vi "边沿计数_事件导出.vi"() -> ()   [LabVIEW 2013]
doc: "This example demonstrates how to count the pulse's edges."
uses:
  <userlib>/ArtDAQ/_SubVI/ArtDAQ_CreateCICountEdgesChan.vi
  <userlib>/ArtDAQ/_SubVI/ArtDAQ_CfgSampClkTiming.vi
  <userlib>/ArtDAQ/_SubVI/ArtDAQ_Read Counter U32 NSamp.vi
panel:
  in  "输出端口":string="Dev1/CTR0"
  in  "脉冲输出极性":i32(ring)=10095 items=["高电平"=10095, "低电平"=10096]
  in  "反转空闲状态":i32(ring)=10192 items=["高"=10192, "低"=10214]
  in  "输出方式":i32(ring)=10265 items=["脉冲方式"=10265, "反转方式"=10307]
  in  "每通道点数":i32=100
  in  "采样速率":dbl=1000.0 format="%#_13g"
  in  "时钟源":string="/Dev1/PFI3"
  in  "计数器":string="Dev1/CTR0"
  out "数据":u32[](array[numeric])
  in  "停止":bool
  out "错误输出":errorcluster
  # "通道属性"
  # "输出事件"
  # "定时"
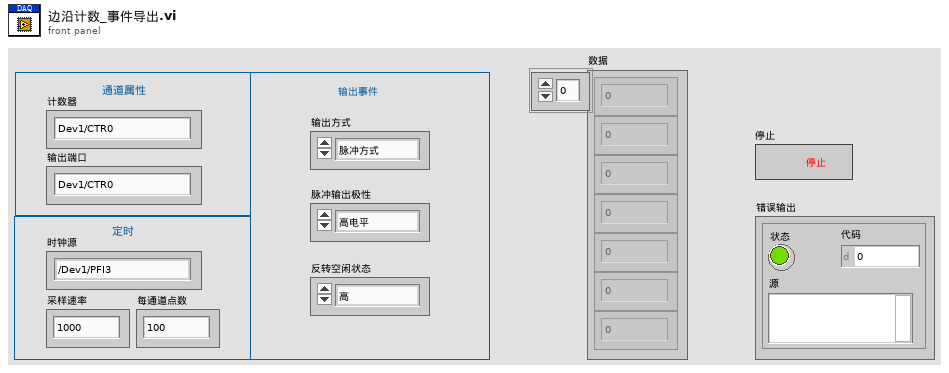
[diagram p1: front panel]
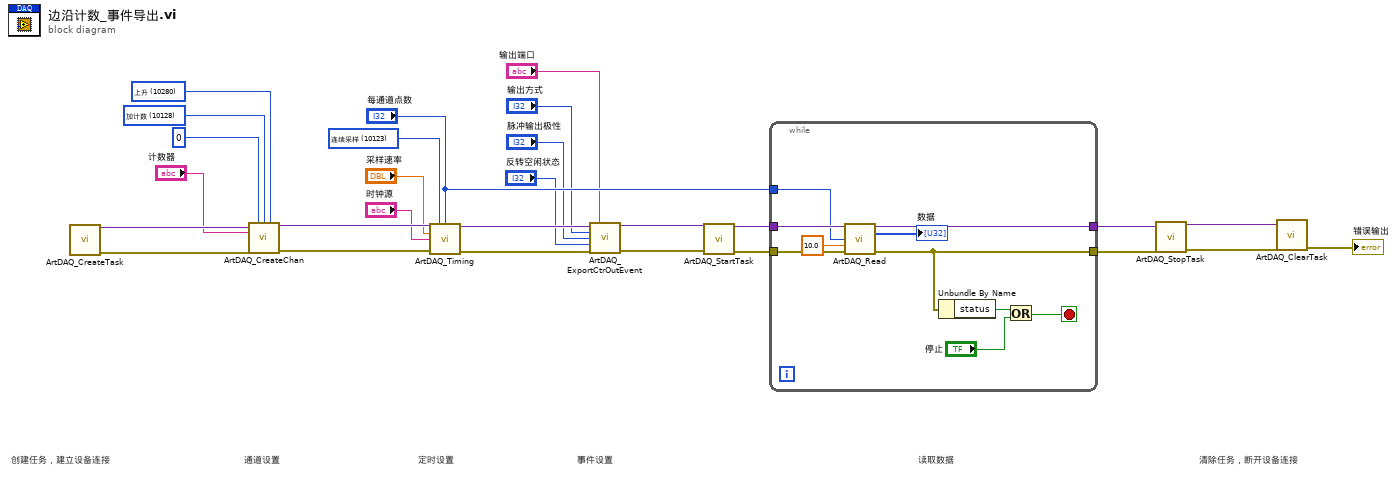
[diagram p0: block diagram]
diagram:
  w10 = 10123 items=["有限点采样"=10178, "连续采样"=10123] ("采样模式")
  w23 = 10280 items=["上升"=10280, "下降"=10171] ("计数边沿")
  w24 = 10128 items=["加计数"=10128, "减计数"=10124, "外部控制"=10326] ("计数方式")
  # "清除任务，断开设备连接"
  # "读取数据"
  # "事件设置"
  # "定时设置"
  # "通道设置"
  # "创建任务，建立设备连接"
  n1 = call <userlib>:"ArtDAQ_CreateTask.vi"() -> ("任务句柄"=w27:variant, "错误输出"=w26:errorcluster)  [unwired: 14 in]
  n2 = call-poly <userlib>:"ArtDAQ_CreateChan.vi"("任务句柄"=w27, "初始计数"=u32 0 ("InitialCount"), "计数方向"=w24, "边沿"=w23, "计数器"="计数器", "错误输入"=w26) -> ("任务句柄"=w14:variant, "错误输出"=w13:errorcluster)  [unwired: 8 in]
  n3 = call-poly <userlib>:"ArtDAQ_Timing.vi"("任务句柄"=w14, "采样模式"=w10, "每通道采样数"="每通道点数", "采样率"="采样速率", "源"="时钟源", "错误输入"=w13) -> ("任务句柄"=w5:variant, "错误输出"=w8:errorcluster)  [unwired: 8 in]
  n4 = call <userlib>:"ArtDAQ_ExportCtrOutEvent.vi"("任务句柄"=w5, "输出接线端"="输出端口", "输出方式"="输出方式", "脉冲极性"="脉冲输出极性", "反转空闲状态"="反转空闲状态", "ErrorInput"=w8) -> ("任务句柄"=w6:variant, "ErrorOutput"=w7:errorcluster)  [unwired: 8 in]
  n5 = call <userlib>:"ArtDAQ_StartTask.vi"("任务句柄"=w6, "错误输入"=w7) -> ("任务句柄"=w16:variant, "错误输出"=w15:errorcluster)  [unwired: 12 in]
  n6 = while {
    tunnel: [w37] -> w21
    tunnel: [w33] -> w19
    tunnel: w16 -> [w36]
    tunnel: w15 -> [w35]
    tunnel: "每通道点数" -> [w29]
    stop <- w30 stop-if-true
    n7 = call-poly <userlib>:"ArtDAQ_Read.vi"("任务句柄"=w36, "每通道采样数"=w29, "超时s"=10.0 ("Timeout"), "错误输入"=w35) -> ("任务句柄"=w37:variant, "数据"=→"数据":u32[], "错误输出"=w33:errorcluster)  [unwired: 9 in]
    n8 = Unbundle By Name(w33) -> ("status"=w32:bool)
    n9 = Or(x=w32, y="停止") -> (x .or. y?=w30:bool)
  }
  n10 = call <userlib>:"ArtDAQ_StopTask.vi"("任务句柄"=w21, "错误输入"=w19) -> ("任务句柄"=w20:variant, "错误输出"=w18:errorcluster)  [unwired: 12 in]
  n11 = call <userlib>:"ArtDAQ_ClearTask.vi"("任务句柄"=w20, "错误输入"=w18) -> ("错误输出"=→"错误输出":errorcluster)  [unwired: 13 in]
